vi "Update.vi"(11 "服务器信息":T1={"host"="27.154.58.30", "port"=8020, "user"="std", "password"="std23506", "远端地址"="/微站/室外总磷总氮高压过滤无主板新电路板/一体化微型水质监测站.exe"}) -> ()   [LabVIEW 2016, in "数据传输系统.lvlib" / "update.lvlib"]
uses:
  update.lvlib
panel:
  out "已下载大小":sgl format="%.2f MB"
  out "滑动杆":dbl(slide) scale=0.0..100.0
  in  "取消按钮":bool
  out "last status string":string caption="最近状态字符串"
  out "command":string caption="命令"
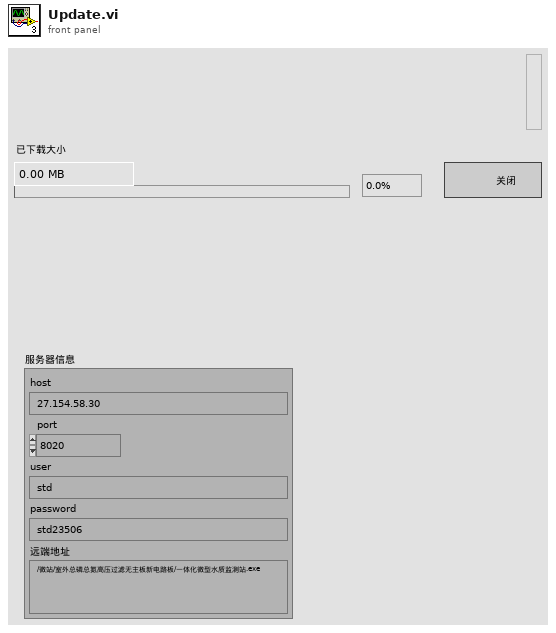
[diagram p1: front panel]
types:
  T1 = cluster{"host":string, "port":u16, "user":string, "password":string, "远端地址":string}
  T2 = cluster{"command":string, "last status string":string, "process":dbl}
  T3 = enum32{"Bad", "Idle", "Run top level", "Running"}
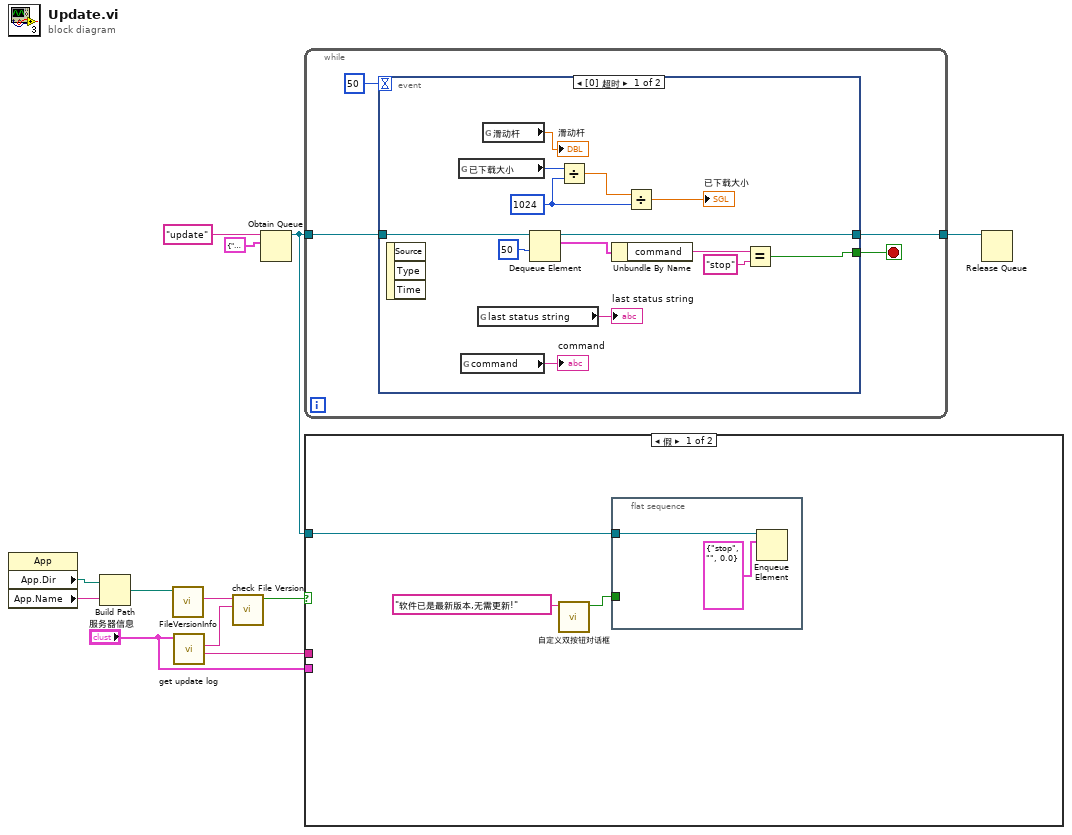
[diagram p0: block diagram]
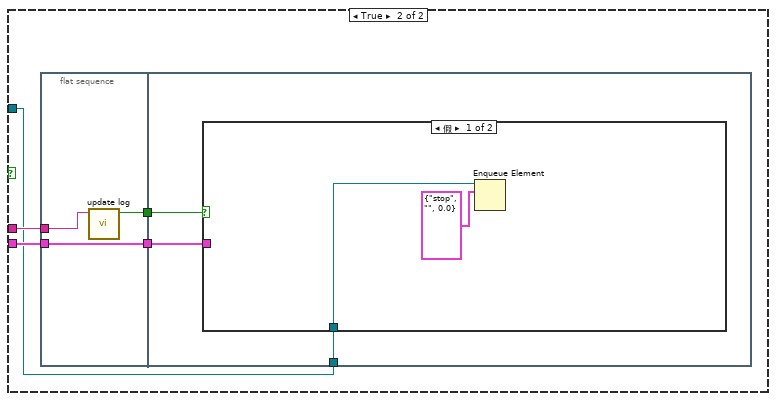
[diagram p2: hidden frame]
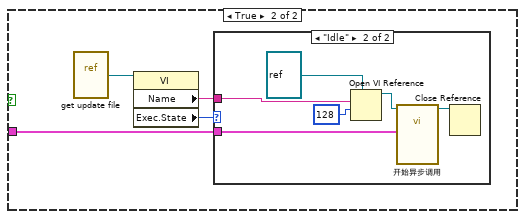
[diagram p3: hidden frame]
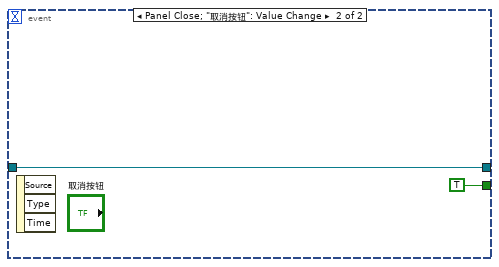
[diagram p5: hidden frame]
diagram:
  n1 = property class="App"() -> ("App.Dir"=w7:path, "App.Name"=w6:string)  [unwired: 2 in, 2 out]
  n2 = Build Path(base path=w7, name or relative path=w6) -> (appended path=w5:path)
  n3 = call <vilib>:"FileVersionInfo.vi"("Application Path in"=w5) -> ("File Version Info"=w1:string)  [unwired: 7 in, 3 out]
  n4 = call "get update log.vi"("服务器信息"="服务器信息") -> ("部分更新日志"=w3:string, "remote File Version"=w8:string)  [unwired: 7 in, 2 out]
  n5 = call "check File Version.vi"("remote File Version Info"=w8, "Local File Version Info"=w1) -> ("new?"=w2:bool)  [unwired: 9 in]
  n6 = Obtain Queue(name (unnamed)="update" ("名称（未命名）"), element data type=T2 {"command"="", "last status string"="", "process"=0.0}) -> (queue out=w4:refnum<queue>)  [unwired: 3 in, 2 out]
  n7 = while {
    tunnel: w4 -> [w14]
    tunnel: [w13] -> w11
    stop <- w15 stop-if-true
    n8 = event shown="[0] 超时" {
      selector: _ -> [_ _]
      dyn-events: _ -> [_ _]
      timeout: 50 -> [_ _]
      tunnel: [w25 TRUE] -> w15
      tunnel: w14 -> [w30 w31]
      tunnel: [w28 w31] -> w13
      event Timeout {
        w18 = i64 1024 ("y")
        n9 = event-data() -> ()  [unwired: 1 in, 3 out]
        n10 = global read "更新全局变量.vi" "已下载大小"() -> (w20:i64)
        n11 = global read "更新全局变量.vi" "command"() -> (→"command":string)
        n12 = global read "更新全局变量.vi" "last status string"() -> (→"last status string":string)
        n13 = global read "更新全局变量.vi" "滑动杆"() -> (→"滑动杆":dbl)
        n14 = Dequeue Element(queue=w30, timeout in ms (-1)=50 ("超时毫秒(-1)")) -> (queue out=w28:refnum<queue>, element=w29:T2)  [unwired: 1 in, 2 out]
        n15 = Divide(x=w20, y=w18) -> (x/y=w19:dbl)
        n16 = Unbundle By Name(w29) -> ("command"=w27:string)
        n17 = Divide(x=w19, y=w18) -> (x/y=→"已下载大小":dbl)
        n18 = Equal?(x=w27, y="stop") -> (x = y?=w25:bool)
      }
      event Panel Close; "取消按钮": Value Change {
        n19 = event-data() -> ()  [unwired: 1 in, 3 out]
      }
    }
  }
  n20 = case shown="假" w2 {
    tunnel: "服务器信息" -> [_ w42]
    tunnel: w3 -> [_ w40]
    tunnel: w4 -> [w35 w38]
    frame False {
      n21 = call "自定义双按钮对话框.vi"("消息"="软件已是最新版本,无需更新!") -> ("输出"=w33:bool)  [unwired: 10 in]
      n22 = flat-sequence {
        tunnel: w35 -> [w37]
        tunnel: w33 -> [_]
        frame #0 {
          n23 = Enqueue Element(queue=w37, element=T2 {"command"="stop", "last status string"="", "process"=0.0} ("元素")) -> ()  [unwired: 2 in, 3 out]
        }
      }
    }
    frame True {
      n24 = flat-sequence {
        tunnel: w42 -> [w45]
        tunnel: [w45] -> w41
        tunnel: w40 -> [w44]
        tunnel: [w43] -> w39
        tunnel: w41 -> [w48]
        tunnel: w39 -> [w47]
        tunnel: w38 -> [w46]
        frame #0 {
          n25 = call "update log.vi"("更新记录"=w44) -> ("check"=w43:bool)  [unwired: 10 in]
        }
        frame #1 {
          n26 = case shown="假" w47 {
            tunnel: w48 -> [_ w51]
            tunnel: w46 -> [w49 _]
            frame False {
              n27 = Enqueue Element(queue=w49, element=T2 {"command"="stop", "last status string"="", "process"=0.0} ("元素")) -> ()  [unwired: 2 in, 3 out]
            }
            frame True {
              n28 = vi-ref "get update file.vi"() -> (w54:refnum<vi>)
              n29 = property class="VI"(reference=w54) -> ("Name"=w53:string, "Exec.State"=w52:T3)  [unwired: 1 in, 2 out]
              n30 = case shown="\"Idle\"" w52 {
                tunnel: w53 -> [_ w60]
                tunnel: w51 -> [_ w56]
                frame "Bad", Default {
                }
                frame "Idle" {
                  n31 = Open VI Reference(type specifier VI Refnum (for type only)=refnum<vi> refnum, vi path=w60, options=128 ("选项")) -> (vi reference=w57:refnum<vi>)  [unwired: 3 in, 1 out]
                  n32 = call-by-ref "开始异步调用"(reference=w57, "服务器信息"=w56) -> (reference out=w58:refnum<vi>)  [unwired: 12 in, 1 out]
                  n33 = Close Reference(reference=w58) -> ()  [unwired: 1 in, 1 out]
                }
              }
            }
          }
        }
      }
    }
  }
  n34 = Release Queue(queue=w11) -> ()  [unwired: 2 in, 3 out]
